vi "5052_driver.vi"(0 "State Path":path, 1 "Data Path":path, 3 "SN":string, 4 "T":string, 5 "EFC":string, 6 "SPURS?":bool, 7 "error in":errorcluster, 8 "# Corr":dbl=100.0, 10 "# Avg":dbl=2.0, 12 "Averageing?":bool=TRUE) -> (9 "Carrier PWR":string, 11 "Max. Spur":string, 13 "error out":errorcluster, 14 "1k":string, 15 "10k":string, 16 "20k":string, 17 "100k":string, 18 "1M":string, 19 "10M":string)   [LabVIEW 2023]
panel:
  out "concatenated string":string
  out "String 3":string
  out "String":string
  # "Phasenoise Acquisition Panel"
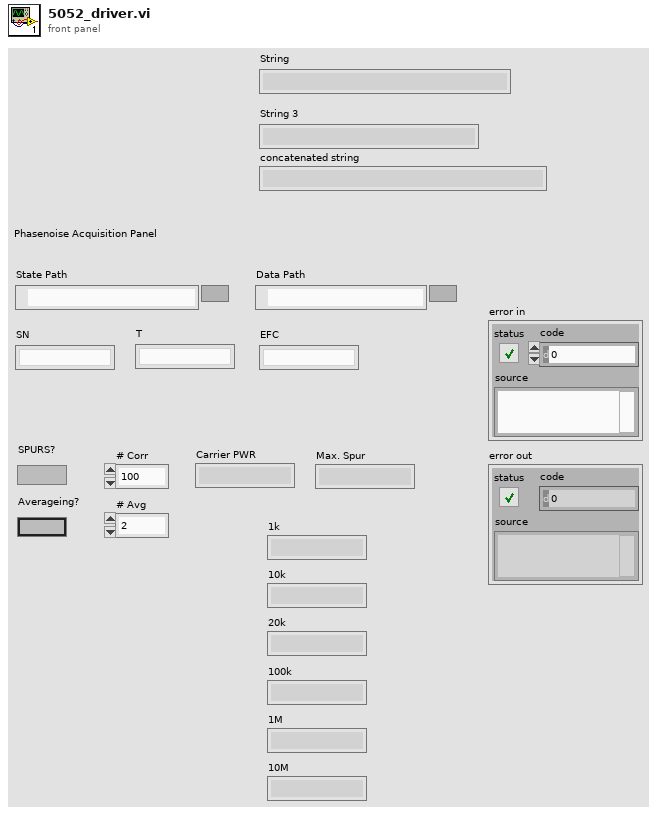
[diagram p1: front panel]
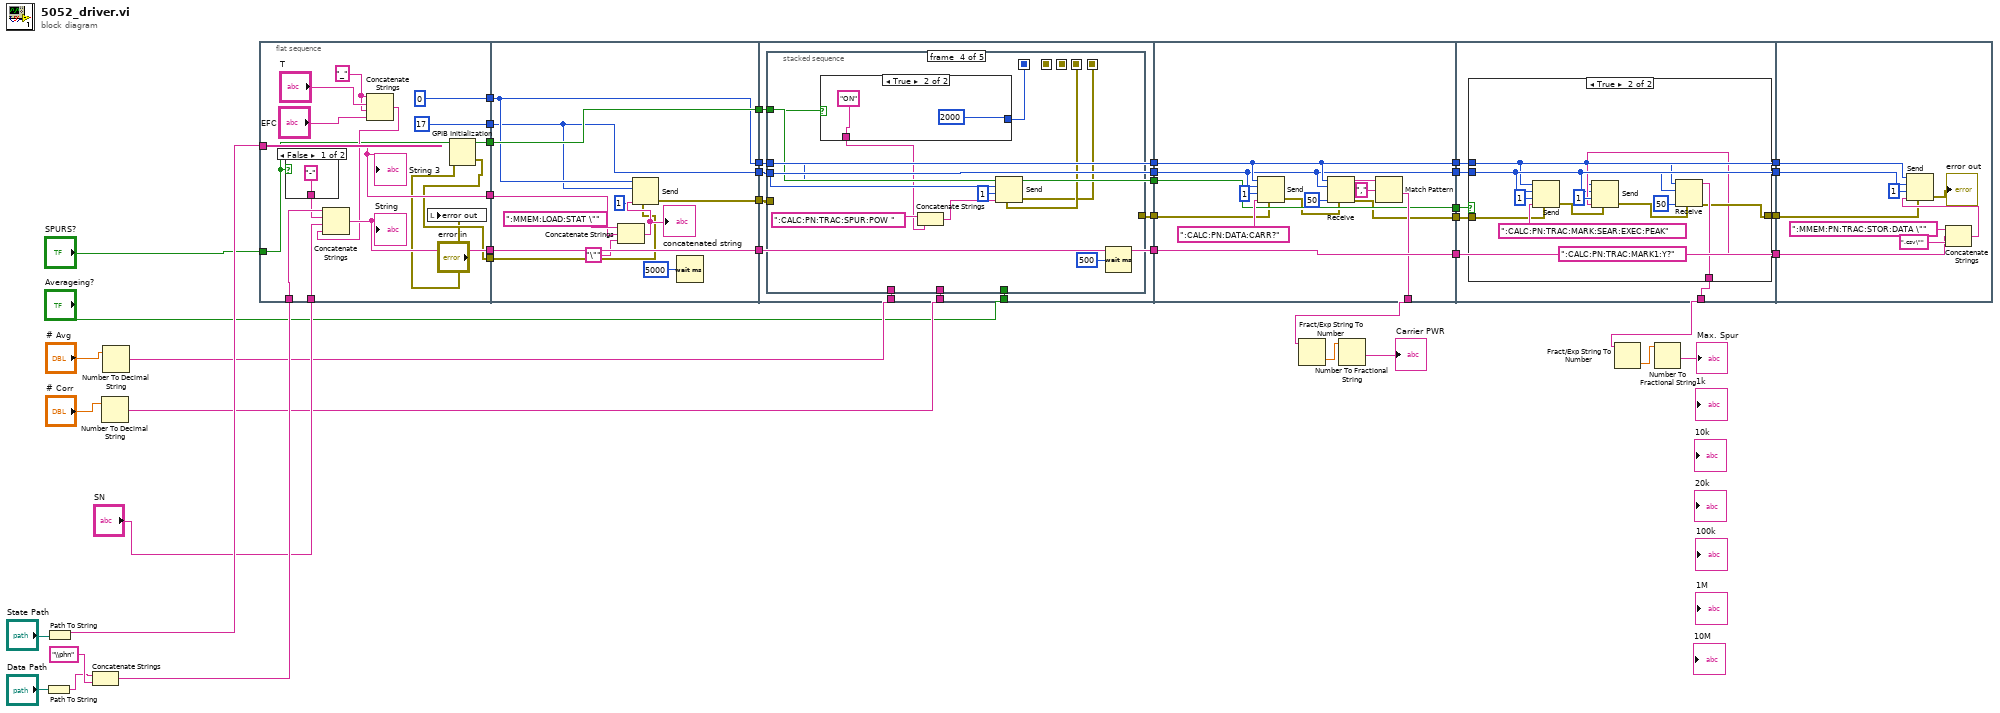
[diagram p0: block diagram]
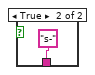
[diagram p2: hidden frame]
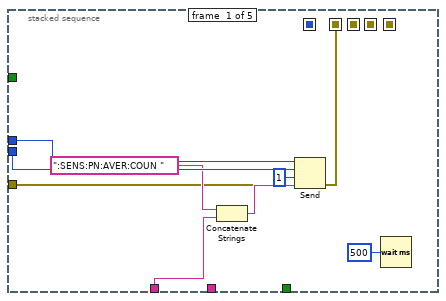
[diagram p3: hidden frame]
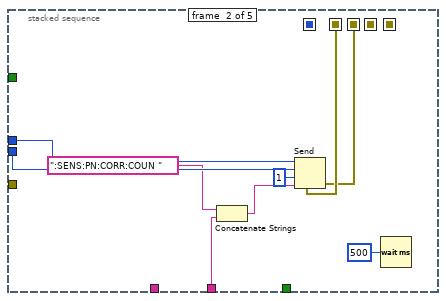
[diagram p4: hidden frame]
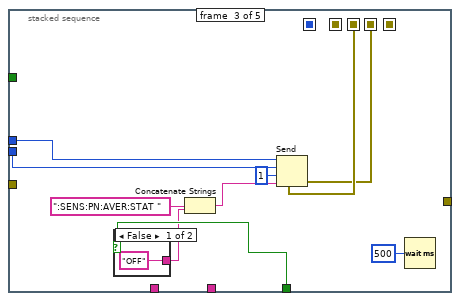
[diagram p5: hidden frame]
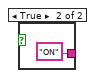
[diagram p6: hidden frame]
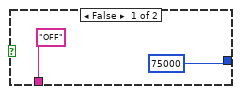
[diagram p7: hidden frame]
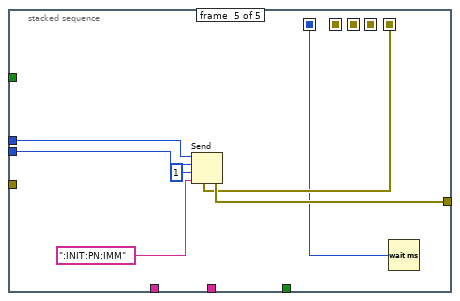
[diagram p8: hidden frame]
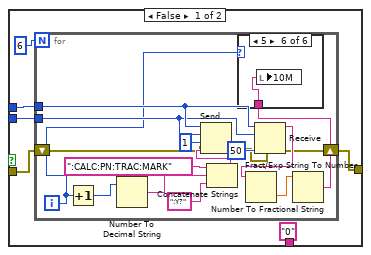
[diagram p9: hidden frame]
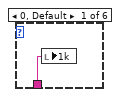
[diagram p10: hidden frame]
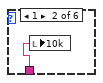
[diagram p11: hidden frame]
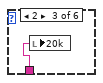
[diagram p12: hidden frame]
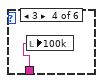
[diagram p13: hidden frame]
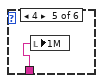
[diagram p14: hidden frame]
diagram:
  n1 = Path To String(path="Data Path") -> (string=w16:string)
  n2 = Path To String(path="State Path") -> (string=w14:string)
  n3 = Concatenate Strings(w16, "\\phn" ("string")) -> (w15:string)
  n4 = Number To Decimal String(number="# Corr") -> (decimal integer string=w10:string)  [unwired: 1 in]
  n5 = Number To Decimal String(number="# Avg") -> (decimal integer string=w11:string)  [unwired: 1 in]
  n6 = flat-sequence {
    tunnel: w14 -> [w55]
    tunnel: w15 -> [w57]
    tunnel: [w55] -> w44
    tunnel: [w56] -> w43
    tunnel: "SPURS?" -> [w51]
    tunnel: "SN" -> [w52]
    tunnel: [w51] -> w42
    tunnel: [0 ("bus")] -> w41
    tunnel: [i16 17 ("address")] -> w40
    tunnel: [w46] -> w39
    tunnel: [w62] -> w35
    tunnel: [w61] -> w36
    tunnel: w44 -> [w70]
    tunnel: [w69] -> w37
    tunnel: w43 -> [w69]
    tunnel: w42 -> [w67]
    tunnel: [w67] -> w38
    tunnel: [w66] -> w34
    tunnel: w41 -> [w62]
    tunnel: w40 -> [w61]
    tunnel: w39 -> [w63]
    tunnel: [w81] -> w33
    tunnel: [w80] -> w32
    tunnel: [w79] -> w31
    tunnel: "Averageing?" -> [w76]
    tunnel: w38 -> [w75]
    tunnel: w10 -> [w77]
    tunnel: w11 -> [w78]
    tunnel: w37 -> [w79]
    tunnel: w36 -> [w80]
    tunnel: w35 -> [w81]
    tunnel: [w75] -> w30
    tunnel: w34 -> [w74]
    tunnel: [w73] -> w29
    tunnel: w33 -> [w144]
    tunnel: w32 -> [w143]
    tunnel: [w144] -> w28
    tunnel: [w143] -> w27
    tunnel: w31 -> [w146]
    tunnel: [w146] -> w26
    tunnel: [w140] -> w7
    tunnel: w30 -> [w139]
    tunnel: [w139] -> w25
    tunnel: [w137] -> w24
    tunnel: w29 -> [w135]
    tunnel: w28 -> [w151]
    tunnel: [w151] -> w23
    tunnel: w27 -> [w150]
    tunnel: [w150] -> w22
    tunnel: w26 -> [w153]
    tunnel: [w153] -> w21
    tunnel: w25 -> [w152]
    tunnel: [w149] -> w5
    tunnel: w24 -> [w148]
    tunnel: [w147] -> w20
    tunnel: w23 -> [w200]
    tunnel: w22 -> [w199]
    tunnel: w21 -> [w197]
    tunnel: w20 -> [w195]
    frame #0 {
      w50 = "_" ("string")
      n7 = case shown="False" w51 {
        tunnel: ["-" "s-"] -> w54
        frame False {
        }
        frame True {
        }
      }
      n8 = Concatenate Strings(w50, "T", w50, "EFC") -> (w53:string)
      n9 = Concatenate Strings(w57, w54, w52, w53) -> (w56:string)
      "String" <- w56
      n10 = local write "error out"("error in") -> ()
      n11 = GPIB Initialization(4:"error in") -> (0:w46:errorcluster)  [unwired: 6 in]
      "String 3" <- w55
    }
    frame #1 {
      n12 = Concatenate Strings(":MMEM:LOAD:STAT \"" ("string"), w70, "\"" ("string")) -> (w72:string)
      "concatenated string" <- w72
      n13 = Send(0:w62, 2:w61, 3:i16 1 ("mode"), 4:w63, 5:w72) -> (8:w66:errorcluster)  [unwired: 2 out]
      n14 = Wait (ms)(milliseconds to wait=u32 5000) -> ()  [unwired: 1 out]
    }
    frame #2 {
      n15 = stacked-sequence {
        seq-local: [w83 _ _ _ _] -> [_ w92 _ _ _]
        seq-local: [_ w91 _ _ _] -> [_ _ w101 _ _]
        seq-local: [_ _ w100 _ _] -> [_ _ _ w116 _]
        seq-local: [_ _ _ w115 _] -> [_ _ _ _ w128]
        seq-local: [_ _ _ w113 _] -> [_ _ _ _ w127]
        tunnel: w81 -> [w90 w99 w109 w122 w133]
        tunnel: w80 -> [w89 w98 w108 w121 w132]
        tunnel: w78 -> [w86 _ _ _ _]
        tunnel: w77 -> [_ w93 _ _ _]
        tunnel: w76 -> [_ _ w106 _ _]
        tunnel: w75 -> [_ _ _ w112 _]
        tunnel: w74 -> [w85 _ _ _ _]
        tunnel: [_ _ _ _ w129] -> w73
        frame #0 {
          n16 = Concatenate Strings(":SENS:PN:AVER:COUN " ("string"), w86) -> (w87:string)
          n17 = Send(0:w90, 2:w89, 3:i16 1 ("mode"), 4:w85, 5:w87) -> (8:w83:errorcluster)  [unwired: 2 out]
          n18 = Wait (ms)(milliseconds to wait=u32 500) -> ()  [unwired: 1 out]
        }
        frame #1 {
          n19 = Concatenate Strings(":SENS:PN:CORR:COUN " ("string"), w93) -> (w96:string)
          n20 = Send(0:w99, 2:w98, 3:i16 1 ("mode"), 4:w92, 5:w96) -> (8:w91:errorcluster)  [unwired: 2 out]
          n21 = Wait (ms)(milliseconds to wait=u32 500) -> ()  [unwired: 1 out]
        }
        frame #2 {
          n22 = case shown="False" w106 {
            tunnel: ["OFF" "ON"] -> w103
            frame False {
            }
            frame True {
            }
          }
          n23 = Concatenate Strings(":SENS:PN:AVER:STAT " ("string"), w103) -> (w107:string)
          n24 = Send(0:w109, 2:w108, 3:i16 1 ("mode"), 4:w101, 5:w107) -> (8:w100:errorcluster)  [unwired: 2 out]
          n25 = Wait (ms)(milliseconds to wait=u32 500) -> ()  [unwired: 1 out]
        }
        frame #3 {
          n26 = case shown="True" w112 {
            tunnel: ["OFF" "ON"] -> w114
            tunnel: [75000 2000] -> w113
            frame False {
            }
            frame True {
            }
          }
          n27 = Concatenate Strings(":CALC:PN:TRAC:SPUR:POW " ("string"), w114) -> (w120:string)
          n28 = Send(0:w122, 2:w121, 3:i16 1 ("mode"), 4:w116, 5:w120) -> (8:w115:errorcluster)  [unwired: 2 out]
          n29 = Wait (ms)(milliseconds to wait=u32 500) -> ()  [unwired: 1 out]
        }
        frame #4 {
          n30 = Send(0:w133, 2:w132, 3:i16 1 ("mode"), 4:w128, 5:":INIT:PN:IMM" ("string")) -> (8:w129:errorcluster)  [unwired: 2 out]
          n31 = Wait (ms)(milliseconds to wait=w127) -> ()  [unwired: 1 out]
        }
      }
    }
    frame #3 {
      n32 = Send(0:w144, 2:w143, 3:i16 1 ("mode"), 4:w135, 5:":CALC:PN:DATA:CARR?" ("string")) -> (8:w136:errorcluster)  [unwired: 2 out]
      n33 = Receive(4:w136, 6:50 ("count"), 8:w143, 9:w144) -> (0:w137:errorcluster, 3:w142:string)  [unwired: 1 in, 2 out]
      n34 = Match Pattern(string=w142, regular expression=",") -> (after substring=w140:string)  [unwired: 1 in, 3 out]
    }
    frame #4 {
      n35 = case shown="True" w152 {
        tunnel: w151 -> [w157 w183]
        tunnel: w150 -> [w156 w182]
        tunnel: ["0" ("data string") w192] -> w149
        tunnel: w148 -> [w154 w190]
        tunnel: [w155 w189] -> w147
        frame False {
          n36 = for {
            N: 6 -> [_]
            tunnel: w157 -> [w175]
            tunnel: w156 -> [w174]
            shift-right: [w164] -> w155
            shift-left: w154 -> [w162]
            i -> [w168]
            n37 = Increment(x=w168) -> (x+1=w169:i32)
            n38 = Number To Decimal String(number=w169) -> (decimal integer string=w170:string)  [unwired: 1 in]
            n39 = Concatenate Strings(":CALC:PN:TRAC:MARK" ("string"), w170, ":Y?") -> (w173:string)
            n40 = Send(0:w175, 2:w174, 3:i16 1 ("mode"), 4:w162, 5:w173) -> (8:w163:errorcluster)  [unwired: 2 out]
            n41 = Receive(4:w163, 6:50 ("count"), 8:w174, 9:w175) -> (0:w164:errorcluster, 3:w167:string)  [unwired: 1 in, 2 out]
            n42 = Fract/Exp String To Number(string=w167) -> (number=w160:dbl)  [unwired: 3 in, 1 out]
            n43 = Number To Fractional String(number=w160) -> (F-format string=w166:string)  [unwired: 3 in]
            n44 = case shown="5" w168 {
              tunnel: w166 -> [w176 w177 w178 w179 w180 w181]
              frame 0, Default {
                n45 = local write "1k"(w176) -> ()
              }
              frame 1 {
                n46 = local write "10k"(w177) -> ()
              }
              frame 2 {
                n47 = local write "20k"(w178) -> ()
              }
              frame 3 {
                n48 = local write "100k"(w179) -> ()
              }
              frame 4 {
                n49 = local write "1M"(w180) -> ()
              }
              frame 5 {
                n50 = local write "10M"(w181) -> ()
              }
            }
          }
        }
        frame True {
          n51 = Send(0:w183, 2:w182, 3:i16 1 ("mode"), 4:w190, 5:":CALC:PN:TRAC:MARK:SEAR:EXEC:PEAK" ("string")) -> (8:w185:errorcluster)  [unwired: 2 out]
          n52 = Send(0:w183, 2:w182, 3:i16 1 ("mode"), 4:w185, 5:":CALC:PN:TRAC:MARK1:Y?" ("string")) -> (8:w186:errorcluster)  [unwired: 2 out]
          n53 = Receive(4:w186, 6:50 ("count"), 8:w182, 9:w183) -> (0:w189:errorcluster, 3:w192:string)  [unwired: 1 in, 2 out]
        }
      }
    }
    frame #5 {
      n54 = Concatenate Strings(":MMEM:PN:TRAC:STOR:DATA \"" ("string"), w197, ".csv\"" ("string")) -> (w198:string)
      n55 = Send(0:w200, 2:w199, 3:i16 1 ("mode"), 4:w195, 5:w198) -> (8:→"error out":errorcluster)  [unwired: 2 out]
    }
  }
  n56 = Fract/Exp String To Number(string=w7) -> (number=w4:dbl)  [unwired: 3 in, 1 out]
  n57 = Number To Fractional String(number=w4) -> (F-format string=→"Carrier PWR":string)  [unwired: 3 in]
  n58 = Fract/Exp String To Number(string=w5) -> (number=w3:dbl)  [unwired: 3 in, 1 out]
  n59 = Number To Fractional String(number=w3) -> (F-format string=→"Max. Spur":string)  [unwired: 3 in]
